vi "Camera Interpreter.vi"() -> (0 "error out":errorcluster, 1 "Overhead Image":T4(plugin-control), 2 "Heading":T1 format="%05.1f", 3 "Boat Location":T2, 4 "Time Elapsed (s)\nSince Last Image":dbl)   [LabVIEW 2011]
uses:
  <vilib>/userdefined/High Color/IMAQdx.ctl
  2-RIO/2 Typedefs/UTM Location.ctl
  2-RIO/2 Typedefs/heading.ctl
  2-RIO/2 Typedefs/indicator LED.ctl
  2-RIO/2 Globals/2 Global.vi
  <vilib>/vision/driver/NI_Vision_Acquisition_Software.lvlib
panel:
  in  "Reset Camera":bool
  in  "Camera Selector":T3="cam0"
  # "(ignore UTM Zone \nand Hemisphere for \nRC boat)"
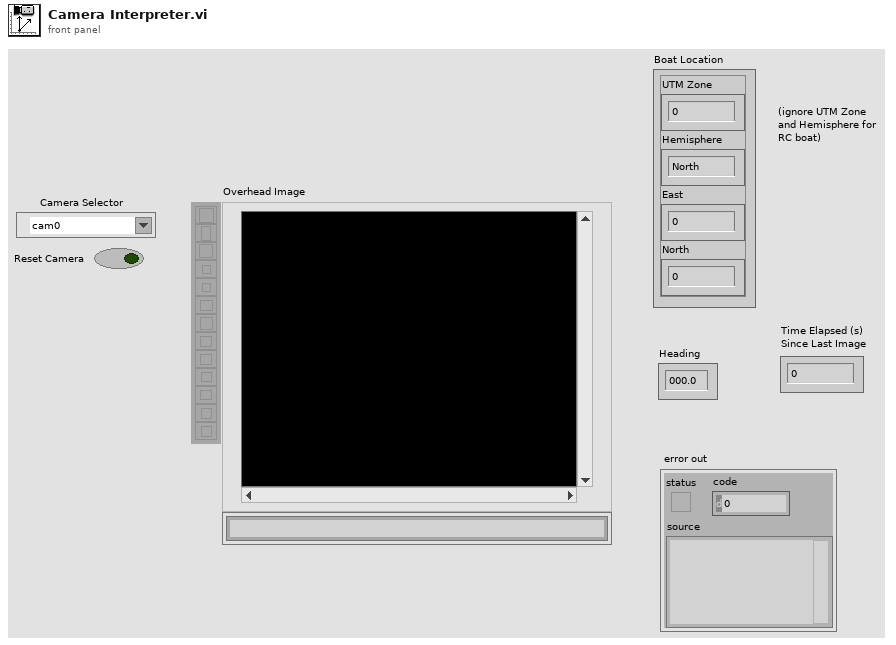
[diagram p1: front panel]
types:
  T1 = typedef "heading.ctl" = dbl
  T2 = typedef "UTM Location.ctl" = cluster{"UTM Zone":dbl, "Hemisphere":enum16{"North", "South"}, "East":dbl, "North":dbl}
  T3 = typedef "IMAQdx.ctl" = refnum<k21>
  T4 = typedef "IMAQ Image.ctl" = refnum<image>
  T5 = typedef "Image Type" = u32
  T6 = typedef "indicator LED.ctl" = bool
  T7 = typedef "generalized sensor status.ctl" = cluster{"Sensor Connected":T6, "Sensor Initialized":T6, "Sensor OK":T6, "Latest Error String":string}
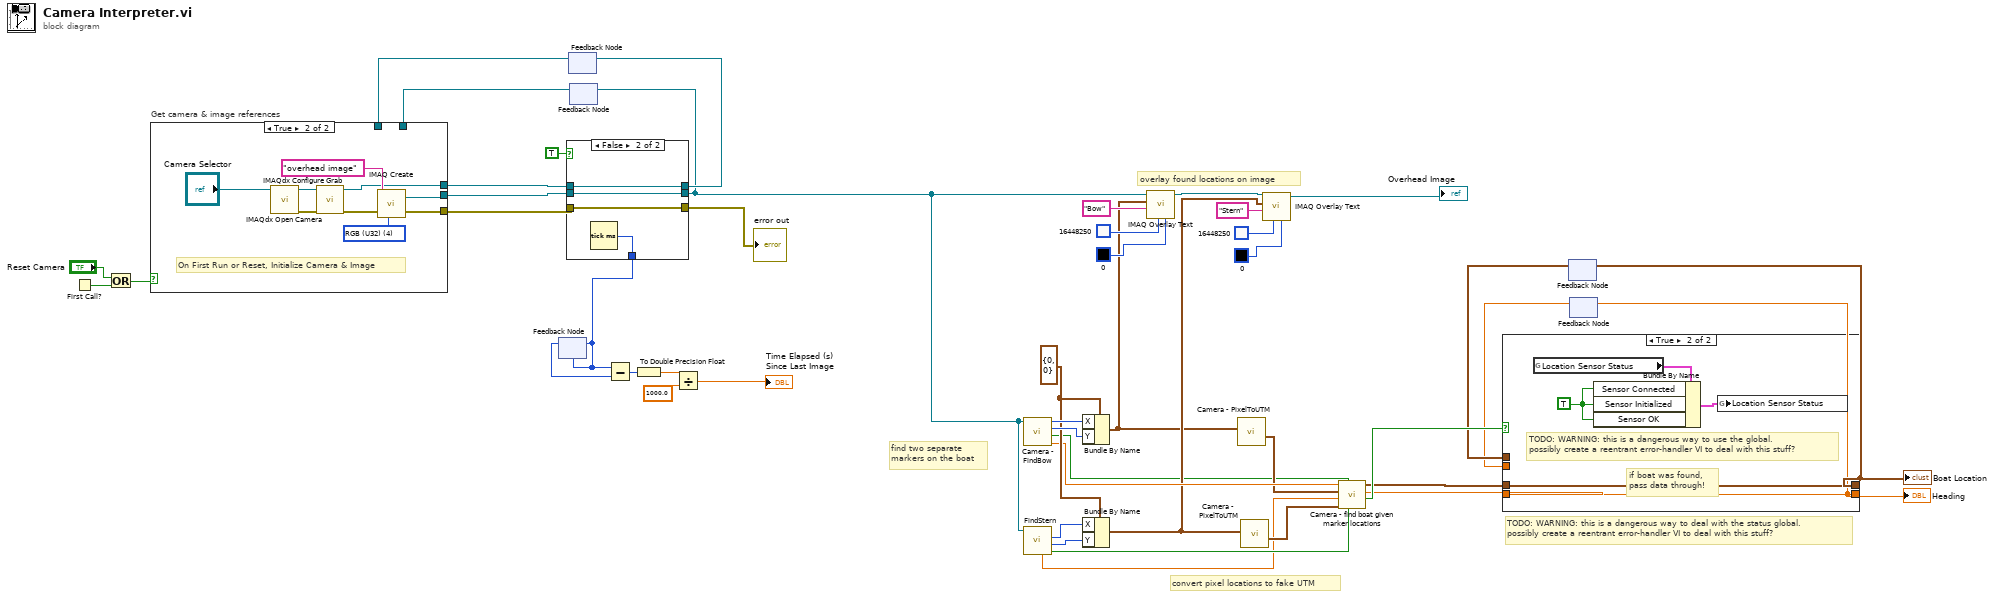
[diagram p0: block diagram]
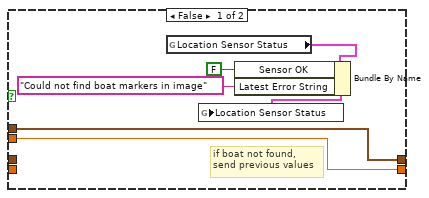
[diagram p2: hidden frame]
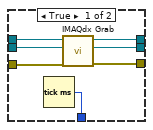
[diagram p3: hidden frame]
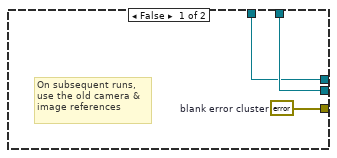
[diagram p4: hidden frame]
diagram:
  w25 = cluster{"X":i32, "Y":i32} {"X"=0, "Y"=0} ("Origin")
  # "TODO: WARNING: this is a dangerous way to deal with the status global. \npossibly create a reentrant error-handler VI to deal with this stuff?"
  # "convert pixel locations to fake UTM"
  # "overlay found locations on image"
  # "find two separate\nmarkers on the boat"
  n1 = First Call?() -> (First Call?: T/F=w45:bool)
  n2 = Or(x="Reset Camera", y=w45) -> (x .or. y?=w38:bool)
  n3 = feedback #1() -> (w39:T3)  [unwired: 1 in]
  n4 = feedback #2() -> (w40:T4)  [unwired: 1 in]
  n5 = case "Get camera & image references" shown="True" w38 {
    tunnel: [w48 w52] -> w44
    tunnel: [w47 w51] -> w43
    tunnel: [w49 w50] -> w42
    tunnel: w40 -> [w49 _]
    tunnel: w39 -> [w48 _]
    frame False {
      w47 = errorcluster {"status"=FALSE, "code"=0, "source"=""}  # blank error cluster
      # "On subsequent runs,\nuse the old camera &\nimage references"
    }
    frame True {
      w54 = T5 4 items=["Grayscale (U8)", "Grayscale (I16)", "Grayscale (SGL)", "Complex (CSG)", "RGB (U32)", "HSL (U32)", "RGB (U64)", "Grayscale (U16)"] ("Image Type")
      # "On First Run or Reset, Initialize Camera & Image"
      n6 = call <vilib>:"IMAQdx Open Camera.vi"("Session In"="Camera Selector") -> ("error out"=w55:errorcluster, "Session Out"=w58:T3)  [unwired: 9 in]
      n7 = call <vilib>:"IMAQdx Configure Grab.vi"("error in"=w55, "Session In"=w58) -> ("error out"=w56:errorcluster, "Session Out"=w52:T3)  [unwired: 8 in]
      n8 = call "IMAQ Create"("Image Name"="overhead image", "Image Type"=w54, "error in (no error)"=w56) -> ("New Image"=w50:T4, "error out"=w51:errorcluster)  [unwired: 2 in]
    }
  }
  n9 = case shown="False" TRUE {
    tunnel: [w65 w67] -> w46
    tunnel: w44 -> [w64 w69]
    tunnel: w43 -> [w63 w67]
    tunnel: w42 -> [w62 w68]
    tunnel: [w61 w68] -> w23
    tunnel: [w60 w69] -> w41
    tunnel: [w59 w66] -> w31
    frame True {
      n10 = Tick Count (ms)() -> (millisecond timer value=w59:u32)
      n11 = call <vilib>:"IMAQdx Grab.vi"("error in"=w63, "Image In"=w62, "Session In"=w64) -> ("error out"=w65:errorcluster, "Image Out"=w61:T4, "Session Out"=w60:T3)  [unwired: 5 in, 1 out]
    }
    frame False {
      n12 = Tick Count (ms)() -> (millisecond timer value=w66:u32)
    }
  }
  "error out" <- w46
  n13 = feedback-in #3(w31) -> ()
  n14 = feedback #3(w31) -> (w36:u32)
  n15 = feedback-in #1(w41) -> ()
  n16 = feedback-in #2(w23) -> ()
  n17 = Subtract(x=w31, y=w36) -> (x-y=w35:u32)
  n18 = To Double Precision Float(number=w35) -> (double precision float=w34:dbl)
  n19 = Divide(x=w34, y=1000.0) -> (x/y=→"Time Elapsed (s)\nSince Last Image":dbl)
  n20 = call "Camera - FindBow.vi"("Refnum in"=w23) -> ("Bow Heading"=w15:T1, "Bow found?"=w9:T6, "bow pixel y"=w28:i32, "bow pixel x"=w29:i32)  [unwired: 7 in]
  n21 = call "FindStern.vi"("Refnum in"=w23) -> ("Stern Found"=w11:T6, "y pixel"=w27:i32, "x pixel"=w26:i32, "Heading"=w8:T1)  [unwired: 6 in, 1 out]
  n22 = Bundle By Name(cluster=w25, "X"=w29, "Y"=w28) -> (w13:cluster{"X":i32, "Y":i32})
  n23 = Bundle By Name(cluster=w25, "X"=w26, "Y"=w27) -> (w14:cluster{"X":i32, "Y":i32})
  n24 = call "IMAQ Overlay Text"("BG Color (Transparent)"=u32 0, "Text Color (black)"=u32 16448250, "String"="Bow", "Origin"=w13, "Image"=w23) -> ("Image Out"=w17:T4)  [unwired: 5 in, 1 out]
  n25 = call "Camera - PixelToUTM.vi"("Found Marker Position in (pixels)"=w13) -> ("UTM Location Out"=w12:T2)  [unwired: 10 in]
  n26 = call "Camera - PixelToUTM.vi"("Found Marker Position in (pixels)"=w14) -> ("UTM Location Out"=w10:T2)  [unwired: 10 in]
  n27 = call "IMAQ Overlay Text"("BG Color (Transparent)"=u32 0, "Text Color (black)"=u32 16448250, "String"="Stern", "Origin"=w14, "Image"=w17) -> ("Image Out"=→"Overhead Image":T4)  [unwired: 5 in, 1 out]
  n28 = call "Camera - find boat given marker locations.vi"("Stern Marker Found"=w11, "Bow Marker Found"=w9, "Stern Marker Location"=w10, "Stern Marker Heading"=w8, "Bow Marker Location"=w12, "Bow Marker Heading"=w15) -> ("Boat Found"=w7:T6, "Heading"=w5:T1, "Boat Location"=w6:T2)  [unwired: 3 in]
  n29 = feedback #4() -> (w3:T2)  [unwired: 1 in]
  n30 = feedback #5() -> (w1:T1)  [unwired: 1 in]
  n31 = case shown="True" w7 {
    tunnel: [w75 w80] -> w4
    tunnel: w6 -> [_ w80]
    tunnel: [w74 w79] -> w2
    tunnel: w5 -> [_ w79]
    tunnel: w3 -> [w75 _]
    tunnel: w1 -> [w74 _]
    frame False {
      # "if boat not found,\nsend previous values"
      n32 = global read "2 Global.vi" "Location Sensor Status"() -> (w73:T7)
      n33 = Bundle By Name(cluster=w73, "Sensor OK"=T6 FALSE, "Latest Error String"="Could not find boat markers in image" ("Error String")) -> (w70:T7)
      n34 = global write "2 Global.vi" "Location Sensor Status"(w70) -> ()
    }
    frame True {
      w76 = T6 TRUE ("Sensor OK")
      # "TODO: WARNING: this is a dangerous way to use the global. \npossibly create a reentrant error-handler VI to deal with this stuff?"
      # "if boat was found, \npass data through!"
      n35 = global read "2 Global.vi" "Location Sensor Status"() -> (w78:T7)
      n36 = Bundle By Name(cluster=w78, "Sensor Connected"=w76, "Sensor Initialized"=w76, "Sensor OK"=w76) -> (w77:T7)
      n37 = global write "2 Global.vi" "Location Sensor Status"(w77) -> ()
    }
  }
  "Boat Location" <- w4
  "Heading" <- w2
  n38 = feedback-in #4(w4) -> ()
  n39 = feedback-in #5(w2) -> ()
